vi "Drag & Drop Run Single.vi"(0 "References In":T1, 3 "error in":errorcluster) -> (6 "References Out":T1, 9 "error out":errorcluster)   [LabVIEW 2015]
uses:
  <vilib>/Utility/miscctls.llb/LVPoint32TypeDef.ctl
panel:
  in  "Coords":T2
  out "Mouse Down?":bool
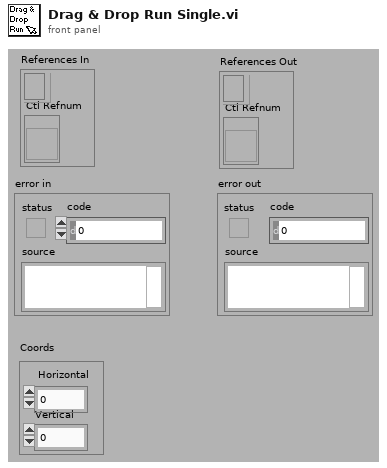
[diagram p1: front panel]
types:
  T1 = cluster{"Event Registration Refnum":refnum<event-registration>, "Ctl Refnum":refnum<vi>}
  T2 = typedef "LVPoint32TypeDef.ctl" = cluster{"Horizontal":i32, "Vertical":i32}
  T3 = typedef "LVPositionTypeDef.ctl" = cluster{"Left":i32, "Top":i32}
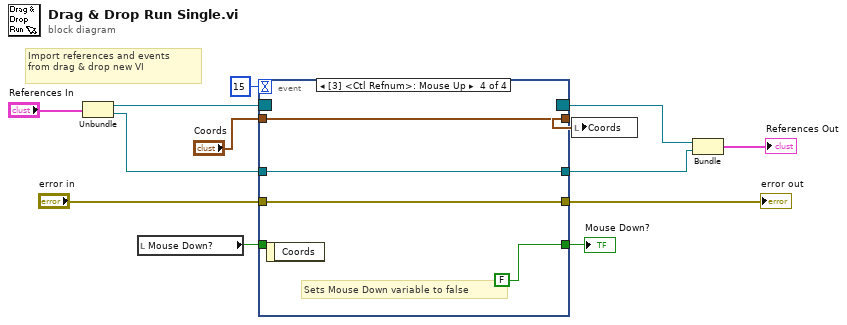
[diagram p0: block diagram]
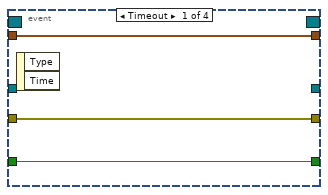
[diagram p2: hidden frame]
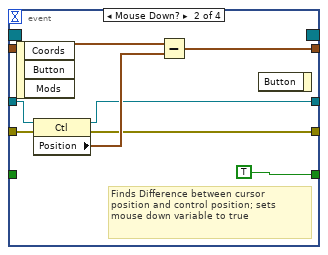
[diagram p3: hidden frame]
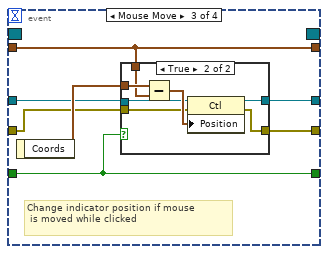
[diagram p4: hidden frame]
diagram:
  # "Import references and events\nfrom drag & drop new VI"
  n1 = Unbundle("References In") -> ("Event Registration Refnum"=w13:refnum<event-registration>, "Ctl Refnum"=w12:refnum<vi>)
  n2 = local read "Mouse Down?"() -> (w3:bool)
  n3 = event shown="[3] <Ctl Refnum>: Mouse Up" {
    selector: w13 -> [_ _ _ _]
    dyn-events: [_ _ _ _] -> w11
    timeout: 15 -> [_ _ _ _]
    tunnel: "Coords" -> [w16 _ w30 w43]
    tunnel: [w16 w23 w30 w43] -> w5
    tunnel: [w14 TRUE ("Boolean") w25 FALSE ("Boolean")] -> w7
    tunnel: [_ w17 w29 w41] -> w10
    tunnel: w12 -> [_ w20 w28 w41]
    tunnel: "error in" -> [w15 w19 w27 w42]
    tunnel: [w15 w18 w26 w42] -> w8
    tunnel: w3 -> [w14 _ w25 _]
    event Timeout {
      n4 = event-data() -> ()  [unwired: 3 out]
    }
    event Mouse Down? {
      # "Finds Difference between cursor\nposition and control position; sets\nmouse down variable to true"
      n5 = event-data() -> ("Coords"=w24:T2)  [unwired: 3 out]
      n6 = property class="Ctl"(reference=w20, error in=w19) -> (reference out=w17:refnum<vi>, error out=w18:errorcluster, "Position"=w21:T3)
      n7 = Subtract(x=w24, y=w21) -> (x-y=w23:T2)
      n8 = event-data() -> ()  [unwired: 1 in, 2 out]
    }
    event Mouse Move {
      # "Change indicator position if mouse\n is moved while clicked"
      n9 = event-data() -> ("Coords"=w31:T2)  [unwired: 1 out]
      n10 = case shown="True" w25 {
        tunnel: w31 -> [_ w40]
        tunnel: w30 -> [_ w39]
        tunnel: [w33 w37] -> w29
        tunnel: w28 -> [w33 w36]
        tunnel: w27 -> [w32 w35]
        tunnel: [w32 w34] -> w26
        frame False {
        }
        frame True {
          n11 = Subtract(x=w40, y=w39) -> (x-y=w38:T2)
          n12 = property class="Ctl"(reference=w36, error in=w35, "Position"=w38) -> (reference out=w37:refnum<vi>, error out=w34:errorcluster)
        }
      }
    }
    event Mouse Up {
      # "Sets Mouse Down variable to false"
      n13 = event-data() -> ()  [unwired: 2 out]
    }
  }
  "error out" <- w8
  "Mouse Down?" <- w7
  n14 = local write "Coords"(w5) -> ()
  n15 = Bundle("Event Registration Refnum"=w11, "Ctl Refnum"=w10) -> (→"References Out":T1)  [unwired: 1 out]
